vi "isSessionActive.vi"(11 "Session in":refnum<class "Session.lvclass">) -> (2 "error out":errorcluster, 3 "Session out":refnum<class "Session.lvclass">)   [LabVIEW 2013, in "MQTT Base.lvlib" / "Session.lvclass"]
uses:
  Session.lvclass
  Session.lvclass/Session.ctl
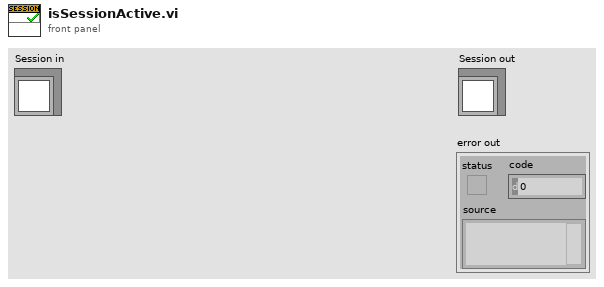
[diagram p1: front panel]
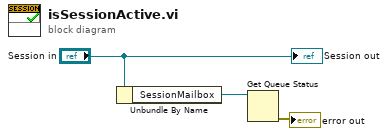
[diagram p0: block diagram]
diagram:
  n1 = Unbundle By Name("Session in") -> ("SessionMailbox"=w3:refnum<queue>)
  n2 = Get Queue Status(queue=w3) -> (error out=→"error out":errorcluster)  [unwired: 2 in, 7 out]
  "Session out" <- "Session in"
